vi "tb_Add Float.vi"() -> ()   [LabVIEW 2011]
panel:
  out "Data Valid":bool[](array[boolean])
  out "Output":sgl[](array[numeric])
  in  "Numeric 2":sgl
  in  "Numeric 1":sgl
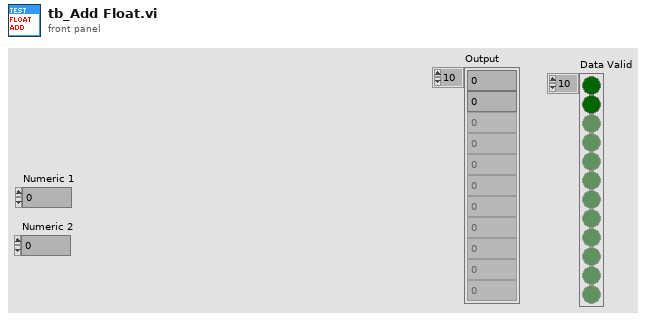
[diagram p1: front panel]
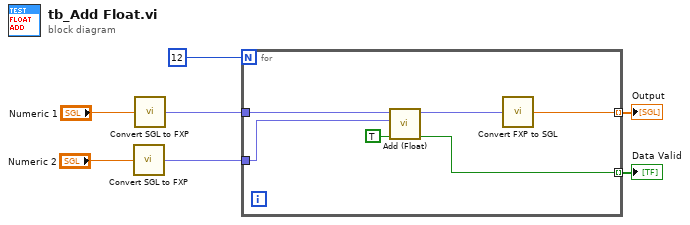
[diagram p0: block diagram]
diagram:
  n1 = call <userlib>:"Convert SGL to FXP.vi"("Input"="Numeric 2") -> ("FXP Output"=w3:fxp<+,32,32>)  [unwired: 14 in]
  n2 = call <userlib>:"Convert SGL to FXP.vi"("Input"="Numeric 1") -> ("FXP Output"=w6:fxp<+,32,32>)  [unwired: 14 in]
  n3 = for {
    N: 12 -> [_]
    tunnel: [w13] -> w1 mode=indexing
    tunnel: w6 -> [w11]
    tunnel: w3 -> [w10]
    tunnel: [w8] -> w2 mode=indexing
    n4 = call <userlib>:"Add (Float).vi"("Input Valid"=TRUE, "b"=w10, "a"=w11) -> ("Output Valid"=w13:bool, "a+b"=w9:fxp<+,32,32>)  [unwired: 7 in]
    n5 = call <userlib>:"Convert FXP to SGL.vi"("FXP Input"=w9) -> ("Output SGL"=w8:sgl)  [unwired: 14 in]
  }
  "Output" <- w2
  "Data Valid" <- w1
